vi "Boolean 2 String.vi"(1 "Boolean":bool) -> (0 "Boolean String":string)   [LabVIEW 2015, in "Configuration.lvlib" / "Section.lvclass"]
doc: "This Vi converts a boolean to string (True/False)."
uses:
  Section.lvclass
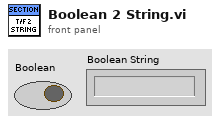
[diagram p1: front panel]
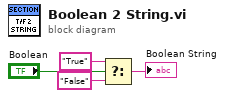
[diagram p0: block diagram]
diagram:
  n1 = Select(t="True", s="Boolean", f="False") -> (s? t:f=→"Boolean String":string)
